vi "send.vi"() -> ()   [LabVIEW 2018]
uses:
  <vilib>/Instr/_visa.llb/VISA Configure Serial Port (Instr).vi
panel:
  in  "路径":path=path "C:/Users/Twsa/Documents/Graduction-Project/send_test.txt"
  out "进度":dbl format="%.2f"
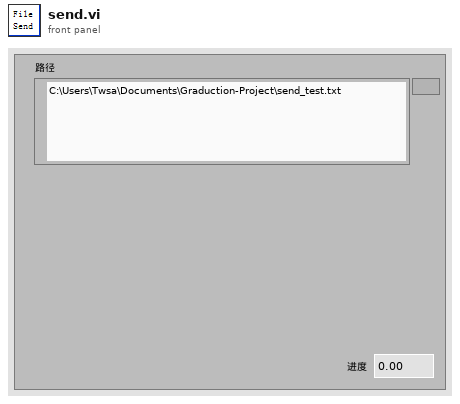
[diagram p1: front panel]
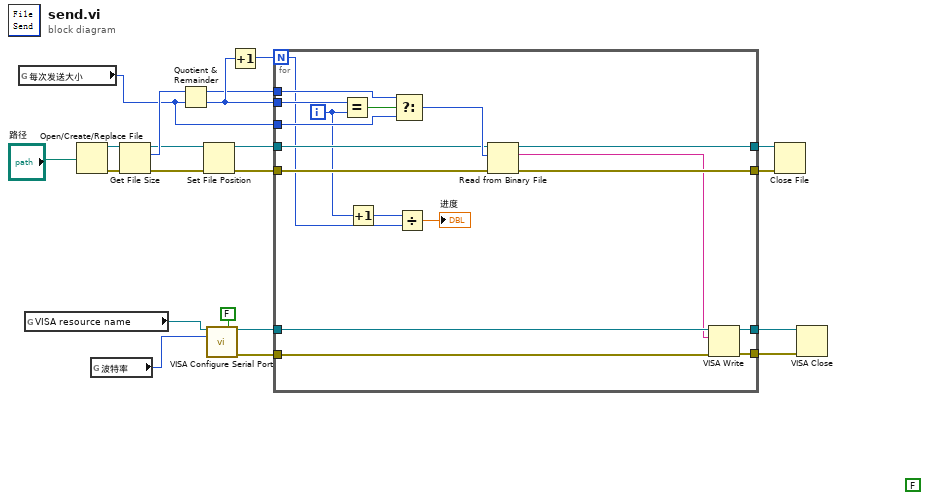
[diagram p0: block diagram]
diagram:
  (unwired) FALSE
  n1 = global read "全局变量.vi" "每次发送大小"() -> (w3:i32)
  n2 = global read "全局变量.vi" "VISA resource name"() -> (w2:refnum<visa-resource-name>)
  n3 = Open/Create/Replace File(file path (use dialog)="路径") -> (refnum out=w14:refnum<file>, error out=w15:errorcluster)  [unwired: 5 in, 1 out]
  n4 = global read "全局变量.vi" "波特率"() -> (w4:u32)
  n5 = Get File Size(file=w14, error in=w15) -> (refnum out=w8:refnum<file>, size (in bytes)=w13:i64, 0:w6:errorcluster)
  n6 = Quotient & Remainder(x=w13, y=w3) -> (x-y*floor(x/y)=w10:i64, floor(x/y)=w12:i64)
  n7 = Set File Position(refnum=w8, error in=w6) -> (refnum out=w7:refnum<file>, error out=w5:errorcluster)  [unwired: 2 in]
  n8 = call-poly "VISA Configure Serial Port"("VISA resource name"=w2, "Enable Termination\nChar (T)"=FALSE ("Enable Termination\nChar (T)"), "baud rate (9600)"=w4) -> ("VISA resource name out"=w21:refnum<visa-resource-name>, "error out"=w20:errorcluster)  [unwired: 11 in]
  n9 = Increment(x=w12) -> (x+1=w11:i64)
  n10 = for {
    N: w11 -> [w24]
    tunnel: w21 -> [w35]
    tunnel: w20 -> [w34]
    tunnel: [w39] -> w17
    tunnel: [w38] -> w16
    tunnel: w7 -> [w27]
    tunnel: w5 -> [w26]
    tunnel: [w37] -> w19
    tunnel: [w36] -> w18
    tunnel: w3 -> [w30]
    tunnel: w12 -> [w33]
    tunnel: w10 -> [w31]
    i -> [w25]
    n11 = Equal?(x=w33, y=w25) -> (x = y?=w32:bool)
    n12 = Increment(x=w25) -> (x+1=w22:i32)
    n13 = Select(t=w31, s=w32, f=w30) -> (s? t:f=w29:i64)
    n14 = Divide(x=w22, y=w24) -> (x/y=→"进度":dbl)
    n15 = Read from Binary File(8:w26, 10:w29, 11:w27) -> (0:w36:errorcluster, 2:w28:string, 3:w37:refnum<file>)  [unwired: 3 in, 1 out]
    n16 = VISA Write(VISA resource name=w35, write buffer=w28, error in (no error)=w34) -> (VISA resource name out=w39:refnum<visa-resource-name>, error out=w38:errorcluster)  [unwired: 1 out]
  }
  n17 = Close File(refnum=w19, error in=w18) -> ()  [unwired: 2 out]
  n18 = VISA Close(VISA resource name=w17, error in (no error)=w16) -> ()  [unwired: 1 out]
